vi "DSDLL Enumerate.vi"(7 "capture devices ring ref":refnum<vi>, 8 "error in":errorcluster, 11 "dsdll session":T1) -> (0 "error out":errorcluster, 2 "version string":string, 3 "dsdll session out":T1)   [LabVIEW 2018, in "DSDLL Virtual Digitizer.lvlib"]
doc: "Enumerates DirectSound capture devices and DSDLL lib version."
uses:
  DSDLL Virtual Digitizer.lvlib
  DSDLL Session.ctl
  dsdll source distribution/dsdll_instance.ctl
  dsdll source distribution/dsdll_device_record.ctl
  DSDLL Process Config.ctl
  DSDLL Data Packet.ctl
  dsdll source distribution/dsdll.lvlib
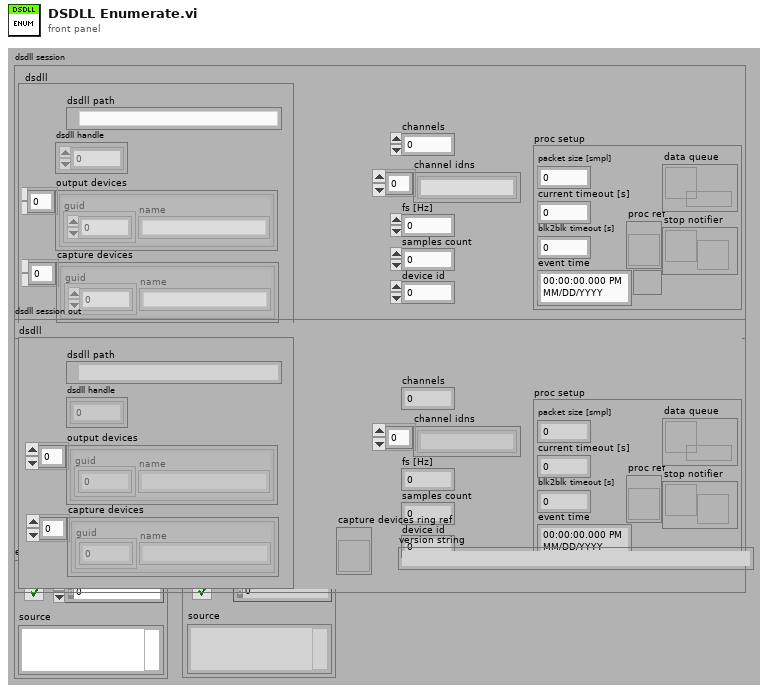
[diagram p1: front panel]
types:
  T1 = typedef "DSDLL Virtual Digitizer.lvlib/DSDLL Session.ctl" = cluster{"dsdll":T2, "channels":i32, "device id":i32, "channel idns":string[], "proc setup":T4, "samples count":i32, "fs [Hz]":dbl}
  T2 = typedef "dsdll.lvlib/dsdll_instance.ctl" = cluster{"dsdll path":path, "dsdll handle":u8[], "output devices":T3[], "capture devices":T3[]}
  T3 = typedef "dsdll.lvlib/dsdll_device_record.ctl" = cluster{"guid":u8[], "name":string}
  T4 = typedef "DSDLL Virtual Digitizer.lvlib/DSDLL Process Config.ctl" = cluster{"packet size [smpl]":i32, "current timeout [s]":dbl, "blk2blk timeout [s]":dbl, "event time":timestamp, "data queue":refnum<queue>, "stop notifier":refnum<notifier>, "proc ref":refnum<vi>}
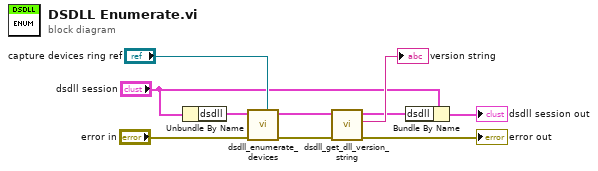
[diagram p0: block diagram]
diagram:
  n1 = Unbundle By Name("dsdll session") -> ("dsdll"=w8:T2)
  n2 = call "dsdll_enumerate_devices.vi"("capture devices ring ref"="capture devices ring ref", "error in"="error in", "dsdll instance in"=w8) -> ("error out"=w9:errorcluster, "dsdll instance out"=w7:T2)  [unwired: 5 in, 2 out]
  n3 = call "dsdll_get_dll_version_string.vi"("error in"=w9, "dsdll instance in"=w7) -> ("error out"=→"error out":errorcluster, "version string"=→"version string":string, "dsdll instance out"=w2:T2)  [unwired: 7 in]
  n4 = Bundle By Name(cluster="dsdll session", "dsdll"=w2) -> (→"dsdll session out":T1)
